vi "XY Graph Special Event Handler Core.vi"(8 "error in (no error)":errorcluster, 9 "Coords":T2, 10 "XYGraph in":T1, 11 "ItemTag":string) -> (0 "error out":errorcluster, 2 "Message":string)   [LabVIEW 2019, in "XY Graph Add-Ons.lvlib"]
uses:
  XY Graph Add-Ons.lvlib
  <vilib>/Utility/miscctls.llb/LVPoint32TypeDef.ctl
  XY Graph Refnum.ctl
  Fit Plot Request Information.ctl
  <vilib>/Utility/miscctls.llb/LVPointDoubleTypeDef.ctl
  Fit Models.ctl
  XY Graph Mouse Click Event Data.ctl
  Plot Editor.lvlib
  Histogram Window.lvlib
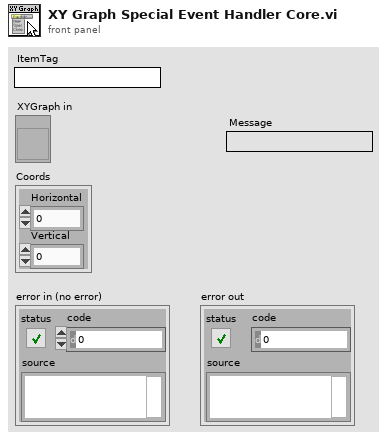
[diagram p1: front panel]
types:
  T1 = typedef "XY Graph Add-Ons.lvlib/XY Graph Refnum.ctl" = refnum<vi>
  T2 = typedef "LVPoint32TypeDef.ctl" = cluster{"Horizontal":i32, "Vertical":i32}
  T3 = typedef "XY Graph Add-Ons.lvlib/XY Graph Mouse Click Event Data.ctl" = cluster{"Multiplot XY Graph":T1, "Mouse Coordinates":T2}
  T4 = typedef "Fit Plot Request Information.ctl" = cluster{"XY Graph Ref":refnum<vi>, "Mouse Coordinates":T5, "Fit Model":T6, "Plot Index":i32}
  T5 = typedef "LVPointDoubleTypeDef.ctl" = cluster{"X":dbl, "Y":dbl}
  T6 = typedef "Fit Models.ctl" = enum16{"Select a Fit Model...", "           Single Peak", "Gaussian", "Asymmetric Gaussian", "Lorentzian", "Asymmetric Lorentzian", "Gaussian/Lorentzian", "Lorentzian/Gaussian", "           Double Peak", "Two Gaussians", "Two Asymmetric Gaussians", "Two H-Connected Gaussians", "Two T-Connected Gaussians", "Two H-Connected Asymmetric Gaussians", "Two T-Connected Asymmetric Gaussians", "           Triple Peak", "Three Gaussians", "Three Asymmetric Gaussians", "              Decays", "Single Exponential", "Two Exponentials", "               ACF", "2D Gaussian ACF", "2D Gaussian + Blinking ACF", "2D Gaussian + Flow ACF", "3D Gaussian ACF", "3D Gaussian + Blinking ACF", "             Multiplot", "2D Gaussian ACF & 2D Gaussian + Flow ACF"}
  T7 = typedef "Plot Style 3.ctl" = cluster{"Plot Style":enum16{"unchanged", "Line", "Symbol", "Line + Symbol", "Histogram", "Histogram + Symbol"}, "Histogram Type":enum16{"unchanged", "Left Bound", "Center", "Right Bound"}, "Line Tickness":enum16{"unchanged", "Thin", "1 pixel", "2 pixel", "3 pixel", "4 pixel", "5 pixel"}, "Line Style":enum16{"unchanged", "Plain", "Long Dash", "Short Dash", "Long-Short Dash", "Long-Short-Short Dash"}, "Point Style":enum16{"unchanged", "None", "Empty Circle", "Filled Circle", "Thick Circle", "Dotted Circle", "Empty Square", "Filled Square", "Thick Square", "Dotted Square", "Small Filled Square", "Dot", "Cross", "Tiny Cross", "Large X", "Small x", "Diamond", "Small Empty Square"}, "Line Color":u32, "Point Color":u32, "Anti-aliased":bool, "Line Color Chooser":enum16{"unchanged", "Color Box", "Color List"}, "Point Color Chooser":enum16{"unchanged", "Color Box", "Color List"}, "Line Color List":string, "Point Color List":string}
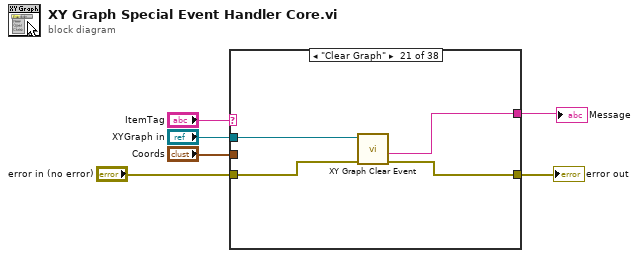
[diagram p0: block diagram]
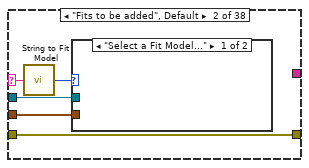
[diagram p3: hidden frame]
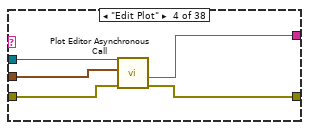
[diagram p6: hidden frame]
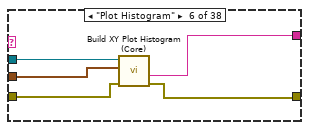
[diagram p8: hidden frame]
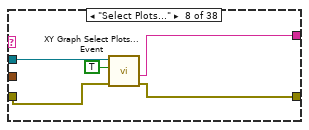
[diagram p10: hidden frame]
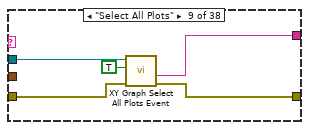
[diagram p11: hidden frame]
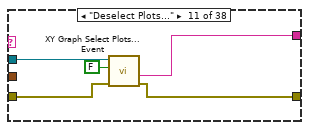
[diagram p13: hidden frame]
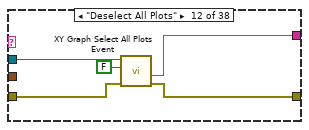
[diagram p14: hidden frame]
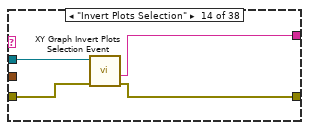
[diagram p16: hidden frame]
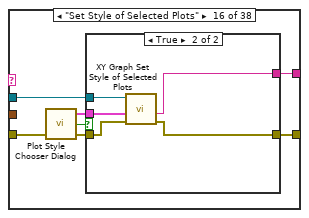
[diagram p18: hidden frame]
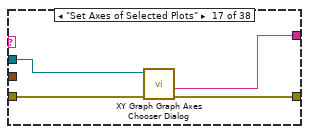
[diagram p20: hidden frame]
diagram:
  n1 = case shown="\"Clear Graph\"" "ItemTag" {
    selector: "ItemTag" -> [_ w9 _ _ _ _ _ _ _ _ _ _ _ _ _ _ _ _ _ _ _ _ _ _ _ _ _ _ _ _ _ _ _ _ _ _ _ _]
    tunnel: "XYGraph in" -> [_ w11 _ w18 _ w24 _ w30 w35 _ w41 w46 _ w51 _ w56 w67 _ w75 w79 w83 _ w87 w93 w98 _ w104 _ w111 _ w118 w123 _ w131 w138 _ w143 w147]
    tunnel: "Coords" -> [_ w10 _ w17 _ w23 _ _ _ _ _ _ _ _ _ _ _ _ w74 _ _ _ w88 _ _ _ _ _ w110 _ _ _ _ w130 w137 _ _ _]
    tunnel: "error in (no error)" -> [w7 w12 w13 w16 w19 w22 w25 w29 w33 w36 w40 w44 w47 w50 w52 w55 w69 w70 w73 w78 w82 w84 w89 w94 w99 w100 w103 w105 w108 w113 w115 w120 w124 w128 w135 w139 w142 w146]
    tunnel: [w7 w12 w13 w15 w19 w21 w25 w27 w31 w36 w38 w42 w47 w49 w52 w54 w68 w70 w71 w77 w81 w84 w86 w92 w97 w100 w102 w105 w107 w113 w116 w121 w124 w127 w134 w139 w141 w145] -> w5
    tunnel: [_ _ _ w14 _ w20 _ w26 w32 _ w37 w43 _ w48 _ w53 w66 _ w72 w76 w80 _ w85 w90 w95 _ w101 _ w106 _ w114 w119 _ w126 w133 _ w140 w144] -> w6
    frame "" {
    }
    frame "Fits to be added", Default {
      (unwired) T4 {"XY Graph Ref"=refnum, "Mouse Coordinates"={"X"=0.0, "Y"=0.0}, "Fit Model"=enum."Select a Fit Model...", "Plot Index"=-1} ("output cluster")
      n2 = call "String to Fit Model.vi"("String"=w9) -> ("Fit Model"=w8:T6)  [unwired: 8 in]
      n3 = case shown="\"Select a Fit Model...\"" w8 {
        tunnel: w11 -> [_ _]
        tunnel: w10 -> [_ _]
        frame "Select a Fit Model..." {
        }
        frame "Gaussian", Default {
        }
      }
    }
    frame "---------" {
    }
    frame "Edit Plot" {
      n4 = call "Plot Editor Asynchronous Call.vi"("error in (no error)"=w16, "Coords"=w17, "XYGraph in"=w18) -> ("Error Out"=w15:errorcluster, "Message"=w14:string)  [unwired: 5 in, 2 out]
    }
    frame "-------------" {
    }
    frame "Plot Histogram" {
      n5 = call "Build XY Plot Histogram (Core).vi"("error in (no error)"=w22, "Mouse Click Coords"=w23, "XYGraph in"=w24) -> ("error out"=w21:errorcluster, "Message"=w20:string)  [unwired: 6 in, 1 out]
    }
    frame "----------------" {
    }
    frame "Select Plots..." {
      n6 = call "XY Graph Select Plots... Event.vi"("Error In"=w29, "Select (T)/Deselect"=TRUE, "XYGraph Ref"=w30) -> ("Error Out"=w27:errorcluster, "Message"=w26:string)  [unwired: 4 in, 3 out]
    }
    frame "Select All Plots" {
      n7 = call "XY Graph Select All Plots Event.vi"("Error In"=w33, "Select (T)/Deselect"=TRUE, "XYGraph Ref"=w35) -> ("Error Out"=w31:errorcluster, "Message"=w32:string)  [unwired: 5 in, 2 out]
    }
    frame "----------------------" {
    }
    frame "Deselect Plots..." {
      n8 = call "XY Graph Select Plots... Event.vi"("Error In"=w40, "Select (T)/Deselect"=FALSE, "XYGraph Ref"=w41) -> ("Error Out"=w38:errorcluster, "Message"=w37:string)  [unwired: 4 in, 3 out]
    }
    frame "Deselect All Plots" {
      n9 = call "XY Graph Select All Plots Event.vi"("Error In"=w44, "Select (T)/Deselect"=FALSE, "XYGraph Ref"=w46) -> ("Error Out"=w42:errorcluster, "Message"=w43:string)  [unwired: 5 in, 2 out]
    }
    frame "-----------------------" {
    }
    frame "Invert Plots Selection" {
      n10 = call "XY Graph Invert Plots Selection Event.vi"("Error In"=w50, "XYGraph Ref"=w51) -> ("Error Out"=w49:errorcluster, "Message"=w48:string)  [unwired: 6 in, 2 out]
    }
    frame "---------------" {
    }
    frame "Set Style of Selected Plots" {
      n11 = call "Plot Style Chooser Dialog.vi"("Error In"=w55) -> ("Plot Style out"=w59:T7, "Cancelled?"=w58:bool, "Error Out"=w57:errorcluster)  [unwired: 6 in]
      n12 = case shown="True" w58 {
        tunnel: w56 -> [_ w65]
        tunnel: w59 -> [_ w64]
        tunnel: w57 -> [w60 w63]
        tunnel: [w60 w62] -> w54
        tunnel: [_ w61] -> w53
        frame False {
        }
        frame True {
          n13 = call "XY Graph Set Style of Selected Plots.vi"("Error In"=w63, "Plot Style"=w64, "XYGraph Ref"=w65) -> ("Error Out"=w62:errorcluster, "Message"=w61:string)  [unwired: 5 in, 2 out]
        }
      }
    }
    frame "Set Axes of Selected Plots" {
      n14 = call "XY Graph Graph Axes Chooser Dialog.vi"("Error In"=w69, "XYGraph Ref"=w67) -> ("Error Out"=w68:errorcluster, "Message"=w66:string)  [unwired: 6 in, 2 out]
    }
    frame "-----------------" {
    }
    frame "Delete Plot" {
      n15 = call "XY Graph Delete Plot Event.vi"("Error In"=w73, "Mouse Click Coordinates"=w74, "XYGraph Ref"=w75) -> ("Error Out"=w71:errorcluster, "Message"=w72:string)  [unwired: 4 in, 3 out]
    }
    frame "Delete Selected Plots" {
      n16 = call "XY Graph Delete Selected Plots Event.vi"("Error In"=w78, "XYGraph Ref"=w79) -> ("Error Out"=w77:errorcluster, "Message"=w76:string)  [unwired: 5 in, 3 out]
    }
    frame "Clear Graph" {
      n17 = call "XY Graph Clear Event.vi"("Error In"=w82, "XYGraph Ref"=w83) -> ("Error Out"=w81:errorcluster, "Message"=w80:string)  [unwired: 7 in, 1 out]
    }
    frame "------------------" {
    }
    frame "Save Plot" {
      n18 = call "XY Graph Save Plot Event.vi"("Error In"=w89, "Mouse Click Coordinates"=w88, "XYGraph Ref"=w87) -> ("Error Out"=w86:errorcluster, "Message"=w85:string)  [unwired: 3 in, 4 out]
    }
    frame "Save Selected Plots" {
      n19 = call "XY Graph Save Selected Plots Event.vi"("Error In"=w94, "Save All Plots? (T)"=FALSE, "XYGraph Ref"=w93) -> ("Error Out"=w92:errorcluster, "Message"=w90:string)  [unwired: 3 in, 4 out]
    }
    frame "Save All Plots" {
      n20 = call "XY Graph Save Selected Plots Event.vi"("Error In"=w99, "Save All Plots? (T)"=TRUE, "XYGraph Ref"=w98) -> ("Error Out"=w97:errorcluster, "Message"=w95:string)  [unwired: 3 in, 4 out]
    }
    frame "------------" {
    }
    frame "Load Plot(s)" {
      n21 = call "XY Graph Load Plot(s) Event.vi"("Error In"=w103, "XYGraph Ref"=w104) -> ("Error Out"=w102:errorcluster, "Message"=w101:string)  [unwired: 4 in, 4 out]
    }
    frame "--------------------------" {
    }
    frame "Transpose Plot" {
      n22 = Bundle(cluster=T3 {"Multiplot XY Graph"=refnum, "Mouse Coordinates"={"Horizontal"=0, "Vertical"=0}} ("Mouse Click Event Data"), "Multiplot XY Graph"=w111, "Mouse Coordinates"=w110) -> (w109:T3)
      n23 = call "XY Graph Transpose Plot Event.vi"("Error In"=w108, "Mouse Click Event Data"=w109) -> ("Error Out"=w107:errorcluster, "Message"=w106:string)  [unwired: 6 in, 2 out]
    }
    frame "--------------------" {
    }
    frame "Add Selected Plots" {
      n24 = call "XY Graph Sum Selected Plots Event.vi"("Error In"=w115, "Add All Plots? (F)"=FALSE, "XYGraph Ref"=w118) -> ("Error Out"=w116:errorcluster, "Message"=w114:string)  [unwired: 3 in, 4 out]
    }
    frame "Add All Plots" {
      n25 = call "XY Graph Sum Selected Plots Event.vi"("Error In"=w120, "Add All Plots? (F)"=TRUE, "XYGraph Ref"=w123) -> ("Error Out"=w121:errorcluster, "Message"=w119:string)  [unwired: 3 in, 4 out]
    }
    frame "---------------------" {
    }
    frame "Single Plot Arithmetic", "y >> f(y) Transform" {
      n26 = Bundle(cluster=T3 {"Multiplot XY Graph"=refnum, "Mouse Coordinates"={"Horizontal"=0, "Vertical"=0}} ("Mouse Click Event Data"), "Multiplot XY Graph"=w131, "Mouse Coordinates"=w130) -> (w129:T3)
      n27 = call "XY Graph Compute Simple Plot Formula Event.vi"("Error In"=w128, "Mouse Click Event Data"=w129) -> ("Error Out"=w127:errorcluster, "Message"=w126:string)  [unwired: 5 in, 3 out]
    }
    frame "(x, y) >> (f, g)(x, y) Transform" {
      n28 = Bundle(cluster=T3 {"Multiplot XY Graph"=refnum, "Mouse Coordinates"={"Horizontal"=0, "Vertical"=0}} ("Mouse Click Event Data"), "Multiplot XY Graph"=w138, "Mouse Coordinates"=w137) -> (w136:T3)
      n29 = call "XY Graph Compute Complex Plot Formula Event.vi"("Error In"=w135, "Mouse Click Event Data"=w136) -> ("Error Out"=w134:errorcluster, "Message"=w133:string)  [unwired: 5 in, 3 out]
    }
    frame "-------------------" {
    }
    frame "Show/Hide Grid" {
      n30 = call "XY Graph Show-Hide Grid Event.vi"("Error In"=w142, "XYGraph in"=w143) -> ("Error Out"=w141:errorcluster, "Message"=w140:string)  [unwired: 8 in]
    }
    frame "Show/Hide Tool Panels" {
      n31 = call "XY Graph Show-Hide Tool Panels Event.vi"("Error In"=w146, "XYGraph in"=w147) -> ("Error Out"=w145:errorcluster, "Message"=w144:string)  [unwired: 8 in]
    }
  }
  "Message" <- w6
  "error out" <- w5
